vi "Create Control (to dir).vi"(8 "error in (no error)":errorcluster, 10 "Target Folder or .ctl":path, 11 "Control in":refnum<class "Control.lvclass">) -> (0 "error out":errorcluster, 3 "Control out":refnum<class "Control.lvclass">)   [LabVIEW 2012, in "Control.lvclass"]
doc: "Create the button control from the object defined with the API modifiers."
uses:
  Control.lvclass
  <userlib>/_OpenG.lib/file/file.llb/Strip Path Extension - Path__ogtk.vi
  <userlib>/_OpenG.lib/file/file.llb/Strip Path - Arrays__ogtk.vi
  <userlib>/_OpenG.lib/file/file.llb/Build Path - Traditional__ogtk.vi
  <userlib>/BitMan/BitMap class/BitMap.lvclass
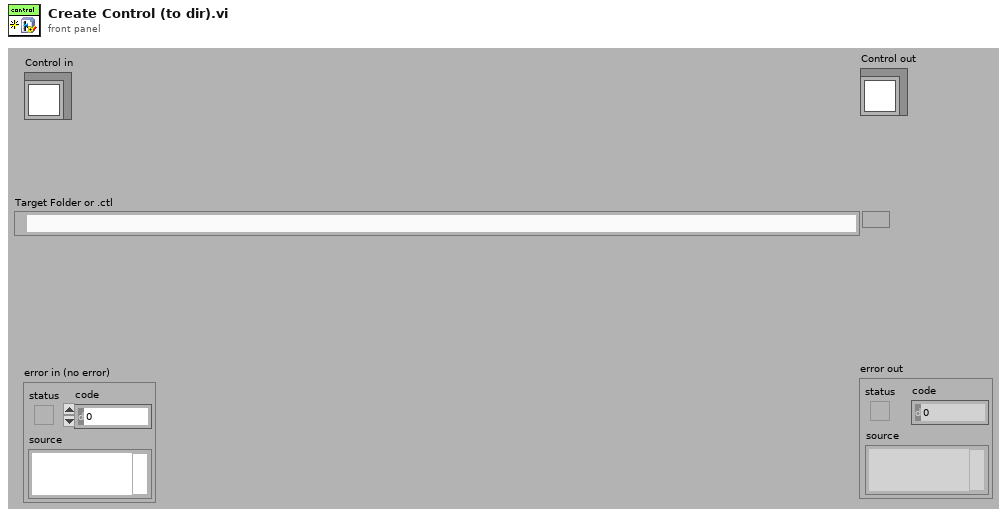
[diagram p1: front panel]
types:
  T1 = typedef "imagedata.ctl" = cluster{"image type":i32, "image depth":i32, "image":u8[], "mask":u8[], "colors":u32[], "Rectangle":cluster{"left":i16, "top":i16, "right":i16, "bottom":i16}}
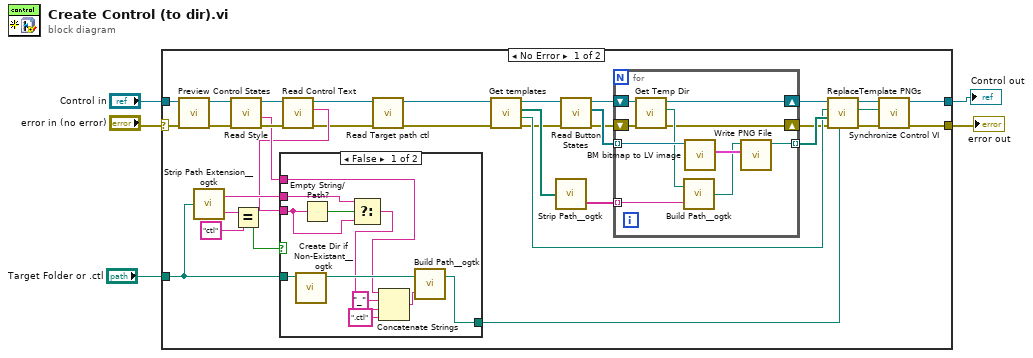
[diagram p0: block diagram]
diagram:
  n1 = case shown="No Error" "error in (no error)" {
    selector: "error in (no error)" -> [w21 w63]
    tunnel: [w27 w63] -> w2
    tunnel: [w28 w62] -> w3
    tunnel: "Control in" -> [w23 w62]
    tunnel: "Target Folder or .ctl" -> [w19 _]
    frame No Error {
      n2 = call-dynamic "Preview Control States.vi"("error in"=w21, "Control in"=w23) -> ("error out"=w20:errorcluster, "Control out"=w22:refnum<class "Control.lvclass">)  [unwired: 8 out]
      n3 = call-poly <userlib>:"Strip Path Extension__ogtk.vi"("path"=w19) -> ("root"=w15:string, "extension"=w18:string)
      n4 = call-dynamic "Read Style.vi"("error in (no error)"=w20, "Control in"=w22) -> ("error out"=w31:errorcluster, "Style name"=w14:string, "Control out"=w37:refnum<class "Control.lvclass">)  [unwired: 7 out]
      n5 = Equal?(x=w18, y="ctl") -> (x = y?=w16:bool)
      n6 = call-dynamic "Read Control Text.vi"("error in (no error)"=w31, "Control in"=w37) -> ("error out"=w10:errorcluster, "Control Text"=w12:string, "Control out"=w11:refnum<class "Control.lvclass">)  [unwired: 7 out]
      n7 = case shown="False" w16 {
        tunnel: w19 -> [w50 w51]
        tunnel: w15 -> [w48 _]
        tunnel: w14 -> [w42 _]
        tunnel: [w40 w51] -> w13
        tunnel: w12 -> [w47 _]
        frame False {
          n8 = call <userlib>:"Create Dir if Non-Existant__ogtk.vi"("Directory Path"=w50) -> ("dup Directory Path"=w43:path)  [unwired: 2 in, 8 out]
          n9 = Empty String/Path?(string/path=w47) -> (empty?=w49:bool)
          n10 = Select(t=w48, s=w49, f=w47) -> (s? t:f=w41:string)
          n11 = Concatenate Strings(w42, "_" ("string"), w41, ".ctl" ("string")) -> (w45:string)
          n12 = call-poly <userlib>:"Build Path__ogtk.vi"("name or relative path"=w45, "base path"=w43) -> ("appended path"=w40:path)
        }
        frame True {
        }
      }
      n13 = call-dynamic "Read Target path ctl.vi"("error in (no error)"=w10, "Control in"=w11) -> ("error out"=w9:errorcluster, "Control out"=w8:refnum<class "Control.lvclass">)  [unwired: 8 out]
      n14 = call-dynamic "Get templates.vi"("error in (no error)"=w9, "Control in"=w8) -> ("error out"=w29:errorcluster, "CTL template"=w36:path, "PNG templates"=w33:path[], "Control out"=w30:refnum<class "Control.lvclass">)  [unwired: 6 out]
      n15 = call-poly <userlib>:"Strip Path__ogtk.vi"("path"=w33) -> ("name"=w32:string[])  [unwired: 1 out]
      n16 = call-dynamic "Read Button States.vi"("error in (no error)"=w29, "Control in"=w30) -> ("error out"=w7:errorcluster, "Button States"=w39:refnum<class "BitMap.lvclass">[], "Control out"=w35:refnum<class "Control.lvclass">)  [unwired: 7 out]
      n17 = for {
        tunnel: [w59] -> w38 mode=indexing
        tunnel: w39 -> [w58] mode=indexing
        shift-right: [w56] -> w34
        shift-left: w35 -> [w57]
        tunnel: w32 -> [w54] mode=indexing
        shift-right: [w52] -> w6
        shift-left: w7 -> [w53]
        n18 = call-dynamic "Get Temp Dir.vi"("error in"=w53, "Control in"=w57) -> ("error out"=w52:errorcluster, "temp directory"=w55:path, "Control out"=w56:refnum<class "Control.lvclass">)  [unwired: 7 out]
        n19 = call-poly <userlib>:"Build Path__ogtk.vi"("name or relative path"=w54, "base path"=w55) -> ("appended path"=w60:path)
        n20 = call <userlib>:"BM bitmap to LV image.vi"("BitMap in"=w58) -> ("LV image data"=w61:T1)  [unwired: 2 in, 8 out]
        n21 = call <vilib>:"Write PNG File.vi"("image data"=w61, "path to PNG file"=w60) -> ("path"=w59:path)  [unwired: 1 in, 8 out]
      }
      n22 = call-dynamic "ReplaceTemplate PNGs.vi"("Control Destination"=w13, "error in"=w6, "States PNGs"=w38, "CTL template"=w36, "Control in"=w34) -> ("error out"=w25:errorcluster, "Control Destination dup"=w24:path, "Control out"=w26:refnum<class "Control.lvclass">)  [unwired: 4 out]
      n23 = call-dynamic "Synchronize Control VI.vi"("error in (no error)"=w25, "Control Destination"=w24, "Control in"=w26) -> ("error out"=w27:errorcluster, "Control out"=w28:refnum<class "Control.lvclass">)  [unwired: 7 out]
    }
    frame Error {
    }
  }
  "error out" <- w2
  "Control out" <- w3
